vi "CASE STRUCTURE IMPLEMETATION .vi"() -> ()   [LabVIEW 2012]
panel:
  out "String 2":string
  in  "String":string
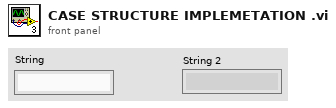
[diagram p1: front panel]
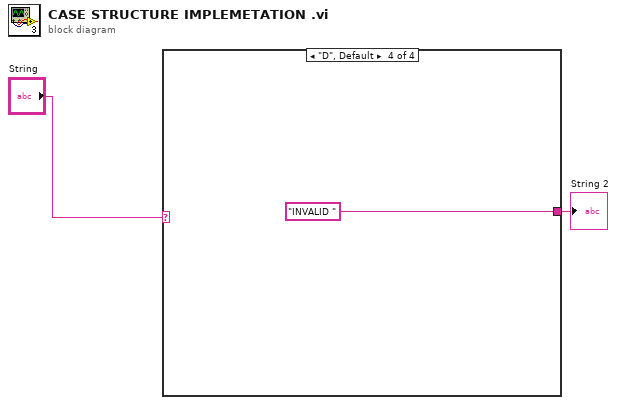
[diagram p0: block diagram]
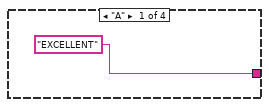
[diagram p2: hidden frame]
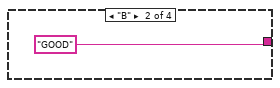
[diagram p3: hidden frame]
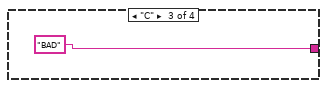
[diagram p4: hidden frame]
diagram:
  n1 = case shown="\"D\", Default" "String" {
    tunnel: ["EXCELLENT" ("String") "GOOD" ("String") "BAD" ("String") "INVALID " ("String")] -> w1
    frame "A" {
    }
    frame "B" {
    }
    frame "C" {
    }
    frame "D", Default {
    }
  }
  "String 2" <- w1
